vi "Excecise 1.vi"() -> ()   [LabVIEW 2013]
panel:
  out "output":dbl
  in  "input":dbl
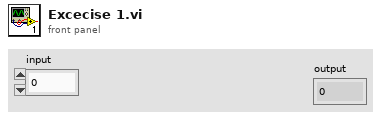
[diagram p1: front panel]
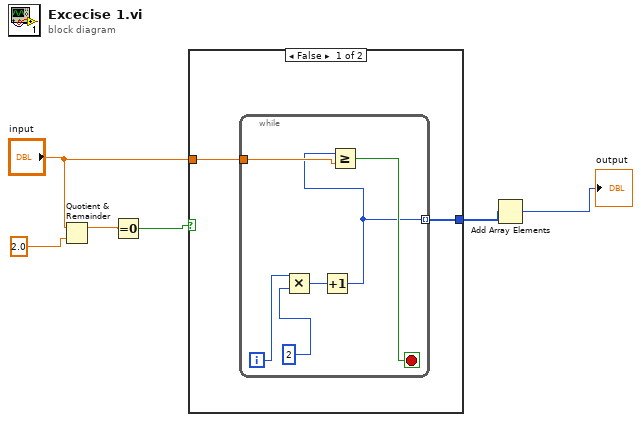
[diagram p0: block diagram]
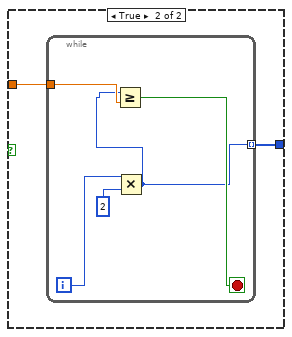
[diagram p2: hidden frame]
diagram:
  n1 = Quotient & Remainder(x="input", y=2.0) -> (x-y*floor(x/y)=w5:dbl)  [unwired: 1 out]
  n2 = Equal To 0?(x=w5) -> (x = 0?=w4:bool)
  n3 = case shown="False" w4 {
    tunnel: "input" -> [w8 w16]
    tunnel: [w7 w15] -> w1
    frame False {
      n4 = while {
        tunnel: w8 -> [w13]
        tunnel: [w9] -> w7 mode=indexing
        i -> [w12]
        stop <- w14 stop-if-true
        n5 = Multiply(x=w12, y=2) -> (x*y=w10:i32)
        n6 = Increment(x=w10) -> (x+1=w9:i32)
        n7 = Greater Or Equal?(x=w9, y=w13) -> (x >= y?=w14:bool)
      }
    }
    frame True {
      n8 = while {
        tunnel: w16 -> [w19]
        tunnel: [w17] -> w15 mode=indexing
        i -> [w20]
        stop <- w18 stop-if-true
        n9 = Multiply(x=w20, y=2) -> (x*y=w17:i32)
        n10 = Greater Or Equal?(x=w17, y=w19) -> (x >= y?=w18:bool)
      }
    }
  }
  n11 = Add Array Elements(numeric array=w1) -> (sum=→"output":i32)
